vi "CUST Get PMU Configuration.vi"(10 "pmuIndex":i32, 11 "pseudoPdcId":i32) -> (0 "function return":i32, 2 "stationName out":string, 3 "pmuconf out":T1)   [LabVIEW 2013, in "C37118-DLL.lvlib"]
doc: "STRONGRIDIEEEC37118DLL_API int __cdecl getPmuConfiguration(pmuConfig* pmuconf, int32_t pseudoPdcId, int32_t pmuIndex);"
uses:
  C37118-DLL.lvlib
  StrongridDLL/StrongridDLL.dll
panel:
  in  "pmuconf":T1
  in  "stationName":string
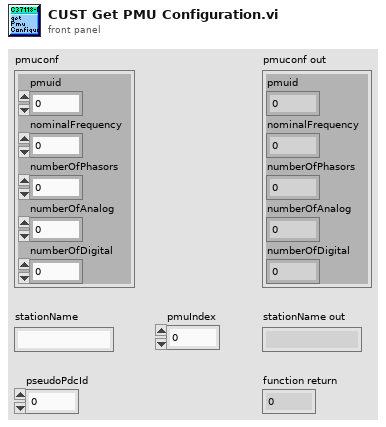
[diagram p1: front panel]
types:
  T1 = cluster{"pmuid":i32, "nominalFrequency":sgl, "numberOfPhasors":i32, "numberOfAnalog":i32, "numberOfDigital":i32}
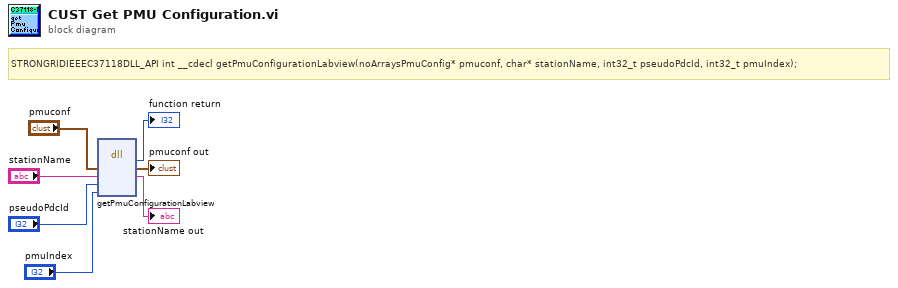
[diagram p0: block diagram]
diagram:
  # "STRONGRIDIEEEC37118DLL_API int __cdecl getPmuConfigurationLabview(noArraysPmuConfig* pmuconf, char* stationName, int32_t pseudoPdcId, int32_t pmuIndex);"
  n1 = dll-call lib="C:/dev/OSS/S3DK/builds/StrongridDLL/StrongridDLL.*" fn="getPmuConfigurationLabview"("pmuconf"="pmuconf", "stationName"="stationName", "pseudoPdcId"="pseudoPdcId", "pmuIndex"="pmuIndex") -> (→"function return":i32, "pmuconf"=→"pmuconf out":T1, "stationName"=→"stationName out":string)  [unwired: 5 in, 2 out]
